vi "SUB_Spent_Seconds.vi"(2 "Current Time ticks":dbl, 3 "start time ticks":dbl) -> (1 "spent time seconds":dbl)   [LabVIEW 2011]
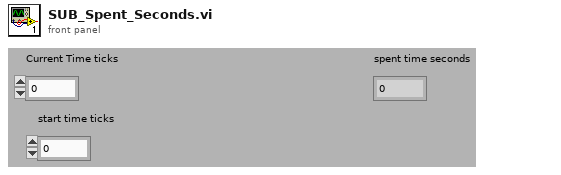
[diagram p1: front panel]
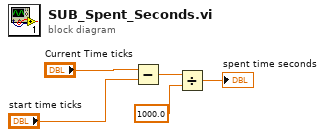
[diagram p0: block diagram]
diagram:
  n1 = Subtract(x="Current Time ticks", y="start time ticks") -> (x-y=w3:dbl)
  n2 = Divide(x=w3, y=1000.0) -> (x/y=→"spent time seconds":dbl)
